vi "BuildStepListFromSteps.vi"(0 "Steps":T2(array[cluster]), 5 "Control Channels":string[](array[string]), 7 "Feedback Channels":string[](array[string]), 9 "AI":string[](array[string])) -> (4 "Step List":string[](array[string]))   [LabVIEW 2015]
panel:
  in  "Step":T1
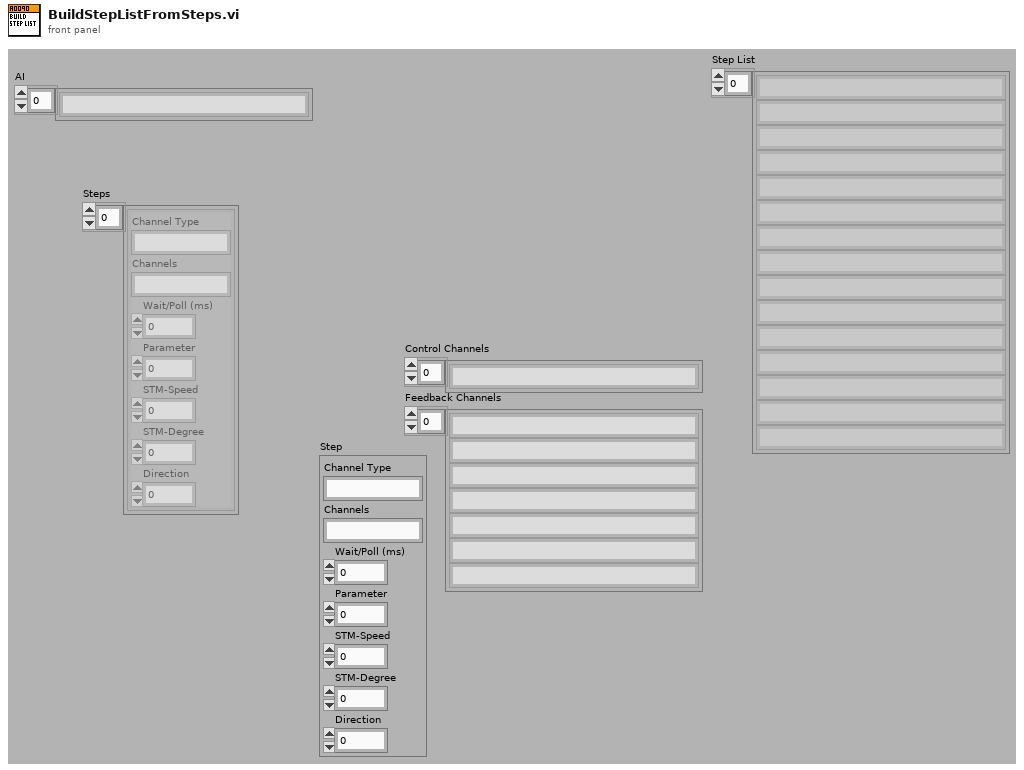
[diagram p1: front panel]
types:
  T1 = cluster{"Channel Type":string, "Channels":string, "Wait/Poll (ms)":u32, "Parameter":u8, "STM-Speed":u8, "STM-Degree":u32, "Direction":u8}
  T2 = cluster{"Channel Type":string, "Channels":string, "Wait/Poll (ms)":u32, "Parameter":u8, "STM-Speed":i32, "STM-Degree":u32, "Direction":u8}[]
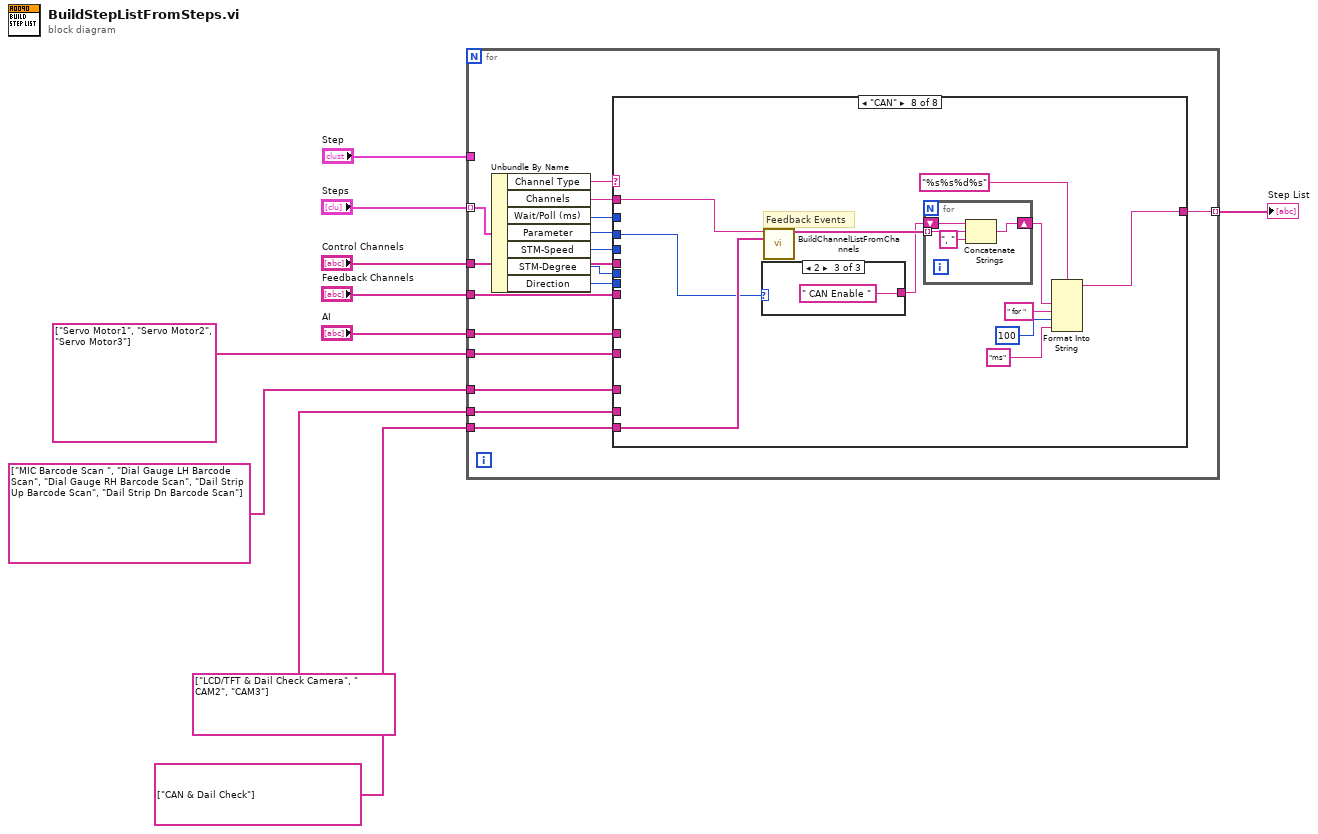
[diagram p0: block diagram]
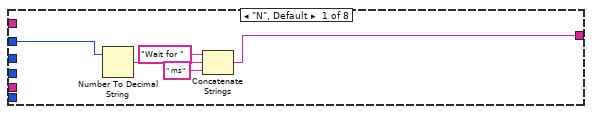
[diagram p2: hidden frame]
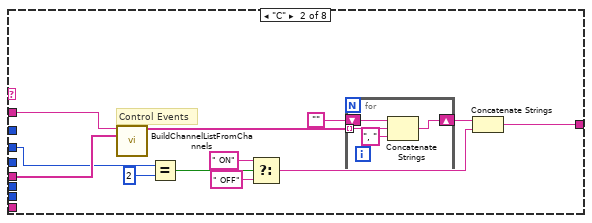
[diagram p3: hidden frame]
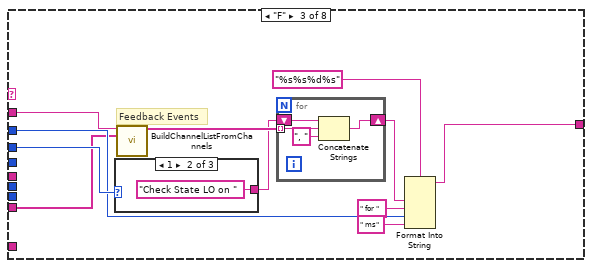
[diagram p4: hidden frame]
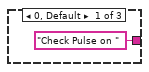
[diagram p5: hidden frame]
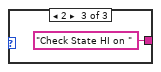
[diagram p6: hidden frame]
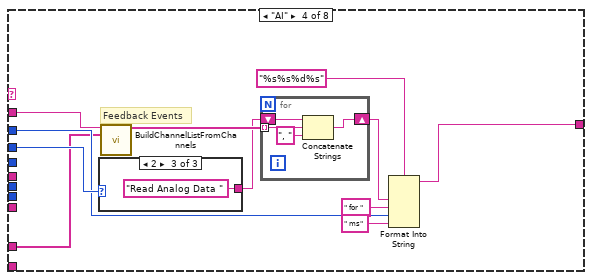
[diagram p7: hidden frame]
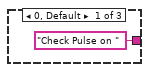
[diagram p8: hidden frame]
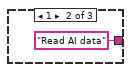
[diagram p9: hidden frame]
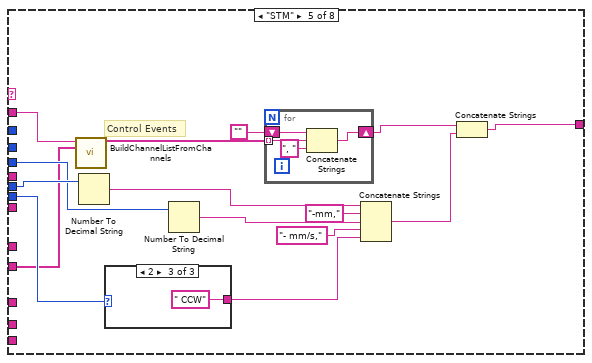
[diagram p10: hidden frame]
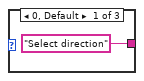
[diagram p11: hidden frame]
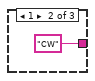
[diagram p12: hidden frame]
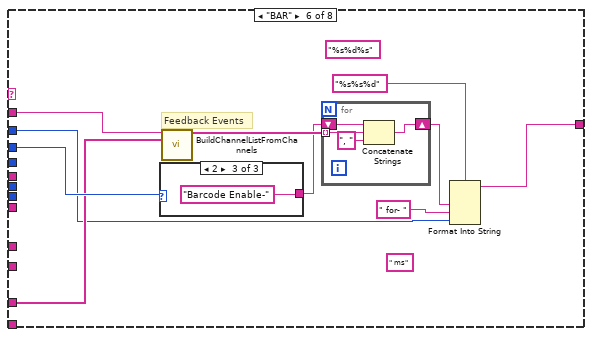
[diagram p13: hidden frame]
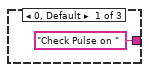
[diagram p14: hidden frame]
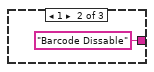
[diagram p15: hidden frame]
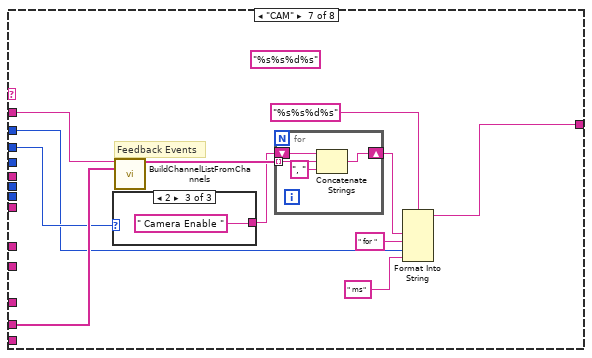
[diagram p16: hidden frame]
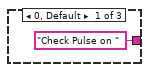
[diagram p17: hidden frame]
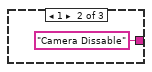
[diagram p18: hidden frame]
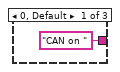
[diagram p19: hidden frame]
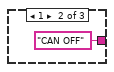
[diagram p20: hidden frame]
diagram:
  n1 = for {
    tunnel: "Steps" -> [w26] mode=indexing
    tunnel: "Control Channels" -> [w22]
    tunnel: "Feedback Channels" -> [w20]
    tunnel: [w19] -> w7 mode=indexing
    tunnel: "Step" -> [_]
    tunnel: "AI" -> [w18]
    tunnel: string[] ["Servo Motor1", "Servo Motor2", "Servo Motor3"] ("Control Channels 2") -> [w14]
    tunnel: string[] ["MIC Barcode Scan ", "Dial Gauge LH Barcode Scan", "Dial Gauge RH Barcode Scan", "Dail Strip Up Barcode Scan", "Dail Strip Dn Barcode Scan"] ("Channel Names (In)") -> [w13]
    tunnel: string[] ["LCD/TFT & Dail Check Camera", " CAM2", "CAM3"] ("Channel Names (In)") -> [w12]
    tunnel: string[] ["CAN & Dail Check"] ("Channel Names (In)") -> [w11]
    n2 = Unbundle By Name(w26) -> ("Channel Type"=w25:string, "Channels"=w23:string, "Wait/Poll (ms)"=w24:u32, "Parameter"=w21:u8, "STM-Speed"=w15:i32, "STM-Degree"=w16:u32, "Direction"=w17:u8)
    n3 = case shown="\"CAN\"" w25 {
      tunnel: w24 -> [w28 _ w53 w69 _ w107 w125 _]
      tunnel: w23 -> [_ w43 w58 w68 w84 w110 w128 w145]
      tunnel: w22 -> [_ w42 _ _ _ _ _ _]
      tunnel: w21 -> [_ w37 w54 w70 _ w111 w126 w144]
      tunnel: w20 -> [_ _ w52 _ _ _ _ _]
      tunnel: [w27 w32 w49 w67 w94 w108 w124 w143] -> w19
      tunnel: w18 -> [_ _ _ w66 _ _ _ _]
      tunnel: w17 -> [_ _ _ _ w95 _ _ _]
      tunnel: w16 -> [_ _ _ _ w93 _ _ _]
      tunnel: w15 -> [_ _ _ _ w90 _ _ _]
      tunnel: w14 -> [_ _ _ _ w85 _ _ _]
      tunnel: w13 -> [_ _ _ _ _ w109 _ _]
      tunnel: w12 -> [_ _ _ _ _ _ w127 _]
      tunnel: w11 -> [_ _ _ _ _ _ _ w146]
      frame "N", Default {
        n4 = Number To Decimal String(number=w28) -> (decimal integer string=w29:string)  [unwired: 1 in]
        n5 = Concatenate Strings("Wait for ", w29, " ms" ("string")) -> (w27:string)
      }
      frame "C" {
        # "Control Events"
        n6 = call "BuildChannelListFromChannels.vi"("Channels (A:B:C:D...) (In)"=w43, "Channel Names (In)"=w42) -> ("Channel List (Out)"=w36:string[])  [unwired: 12 in, 1 out]
        n7 = Equal?(x=w37, y=u8 2) -> (x = y?=w40:bool)
        n8 = Select(t=" ON", s=w40, f=" OFF") -> (s? t:f=w34:string)
        n9 = for {
          tunnel: w36 -> [w47] mode=indexing
          shift-right: [w44] -> w33
          shift-left: "" -> [w45]
          n10 = Concatenate Strings(w45, w47, ", " ("string")) -> (w44:string)
        }
        n11 = Concatenate Strings(w33, w34) -> (w32:string)
      }
      frame "F" {
        # "Feedback Events"
        n12 = case shown="1" w54 {
          tunnel: ["Check Pulse on " "Check State LO on " "Check State HI on "] -> w48
          frame 0, Default {
          }
          frame 1 {
          }
          frame 2 {
          }
        }
        n13 = call "BuildChannelListFromChannels.vi"("Channels (A:B:C:D...) (In)"=w58, "Channel Names (In)"=w52) -> ("Channel List (Out)"=w57:string[])  [unwired: 12 in, 1 out]
        n14 = for {
          tunnel: w57 -> [w65] mode=indexing
          shift-right: [w62] -> w50
          shift-left: w48 -> [w63]
          n15 = Concatenate Strings(w63, w65, ", " ("string")) -> (w62:string)
        }
        n16 = Format Into String(format string="%s%s%d%s", w50, " for " ("input 1"), w53, " ms" ("input 3")) -> (resulting string=w49:string)  [unwired: 2 in, 1 out]
      }
      frame "AI" {
        # "Feedback Events"
        n17 = case shown="2" w70 {
          tunnel: ["Check Pulse on " "Read AI data" "Read Analog Data "] -> w71
          frame 0, Default {
          }
          frame 1 {
          }
          frame 2 {
          }
        }
        n18 = call "BuildChannelListFromChannels.vi"("Channels (A:B:C:D...) (In)"=w68, "Channel Names (In)"=w66) -> ("Channel List (Out)"=w76:string[])  [unwired: 12 in, 1 out]
        n19 = for {
          tunnel: w76 -> [w83] mode=indexing
          shift-right: [w80] -> w72
          shift-left: w71 -> [w81]
          n20 = Concatenate Strings(w81, w83, ", " ("string")) -> (w80:string)
        }
        n21 = Format Into String(format string="%s%s%d%s", w72, " for " ("input 1"), w69, " ms" ("input 3")) -> (resulting string=w67:string)  [unwired: 2 in, 1 out]
      }
      frame "STM" {
        # "Control Events"
        n22 = call "BuildChannelListFromChannels.vi"("Channels (A:B:C:D...) (In)"=w84, "Channel Names (In)"=w85) -> ("Channel List (Out)"=w98:string[])  [unwired: 12 in, 1 out]
        n23 = Number To Decimal String(number=w93) -> (decimal integer string=w92:string)  [unwired: 1 in]
        n24 = case shown="2" w95 {
          tunnel: ["Select direction" "CW" " CCW"] -> w87
          frame 0, Default {
          }
          frame 1 {
          }
          frame 2 {
          }
        }
        n25 = Number To Decimal String(number=w90) -> (decimal integer string=w89:string)  [unwired: 1 in]
        n26 = for {
          tunnel: w98 -> [w105] mode=indexing
          shift-right: [w102] -> w96
          shift-left: "" -> [w103]
          n27 = Concatenate Strings(w103, w105, ", " ("string")) -> (w102:string)
        }
        n28 = Concatenate Strings(w92, "-mm," ("string"), w89, "- mm/s," ("string"), w87) -> (w86:string)
        n29 = Concatenate Strings(w96, w86) -> (w94:string)
      }
      frame "BAR" {
        (unwired) "%s%d%s" ("format string")
        (unwired) " ms" ("input 3")
        # "Feedback Events"
        n30 = case shown="2" w111 {
          tunnel: ["Check Pulse on " "Barcode Dissable" "Barcode Enable-"] -> w112
          frame 0, Default {
          }
          frame 1 {
          }
          frame 2 {
          }
        }
        n31 = call "BuildChannelListFromChannels.vi"("Channels (A:B:C:D...) (In)"=w110, "Channel Names (In)"=w109) -> ("Channel List (Out)"=w115:string[])  [unwired: 12 in, 1 out]
        n32 = for {
          tunnel: w115 -> [w122] mode=indexing
          shift-right: [w119] -> w113
          shift-left: w112 -> [w120]
          n33 = Concatenate Strings(w120, w122, ", " ("string")) -> (w119:string)
        }
        n34 = Format Into String(format string="%s%s%d", w113, " for- " ("input 1"), w107) -> (resulting string=w108:string)  [unwired: 2 in, 1 out]
      }
      frame "CAM" {
        (unwired) "%s%s%d%s" ("format string")
        # "Feedback Events"
        n35 = case shown="2" w126 {
          tunnel: ["Check Pulse on " "Camera Dissable" " Camera Enable "] -> w129
          frame 0, Default {
          }
          frame 1 {
          }
          frame 2 {
          }
        }
        n36 = call "BuildChannelListFromChannels.vi"("Channels (A:B:C:D...) (In)"=w128, "Channel Names (In)"=w127) -> ("Channel List (Out)"=w133:string[])  [unwired: 12 in, 1 out]
        n37 = for {
          tunnel: w133 -> [w140] mode=indexing
          shift-right: [w137] -> w130
          shift-left: w129 -> [w138]
          n38 = Concatenate Strings(w138, w140, ", " ("string")) -> (w137:string)
        }
        n39 = Format Into String(format string="%s%s%d%s", w130, " for " ("input 1"), w125, " ms" ("input 3")) -> (resulting string=w124:string)  [unwired: 2 in, 1 out]
      }
      frame "CAN" {
        # "Feedback Events"
        n40 = case shown="2" w144 {
          tunnel: ["CAN on " "CAN OFF" " CAN Enable "] -> w147
          frame 0, Default {
          }
          frame 1 {
          }
          frame 2 {
          }
        }
        n41 = call "BuildChannelListFromChannels.vi"("Channels (A:B:C:D...) (In)"=w145, "Channel Names (In)"=w146) -> ("Channel List (Out)"=w151:string[])  [unwired: 12 in, 1 out]
        n42 = for {
          tunnel: w151 -> [w158] mode=indexing
          shift-right: [w155] -> w148
          shift-left: w147 -> [w156]
          n43 = Concatenate Strings(w156, w158, ", " ("string")) -> (w155:string)
        }
        n44 = Format Into String(format string="%s%s%d%s", w148, " for " ("input 1"), u32 100 ("input 3"), "ms" ("input 4")) -> (resulting string=w143:string)  [unwired: 2 in, 1 out]
      }
    }
  }
  "Step List" <- w7
